vi "DCPowerlaw4i.vi"() -> ()   [LabVIEW 2011]
panel:
  in  "Temperature Array (K)":dbl[](array[numeric])=[6.0, 7.0, 8.0, 9.0, 10.0, 11.0] format="%#_6p"
  in  "Most Negative Voltage [V]":dbl=-5.0 format="%#.7p"
  in  "Voltage Step [V] 2":dbl=0.01 format="%#_7p"
  in  "Most Positive Voltage [V] 2":dbl=5.0 format="%#.7p"
  out "Temperature [K]":dbl
  out "V vs. Freq. 2":cluster{"Y":dbl[], "Y":dbl[]}[](graph)
  out "V vs. Freq.":cluster{"Y":dbl[], "Y":dbl[]}[](graph)
  in  "Voltage Step [V]":dbl=0.01 format="%#_7p"
  in  "Most Positive Voltage [V]":dbl=5.0 format="%#.7p"
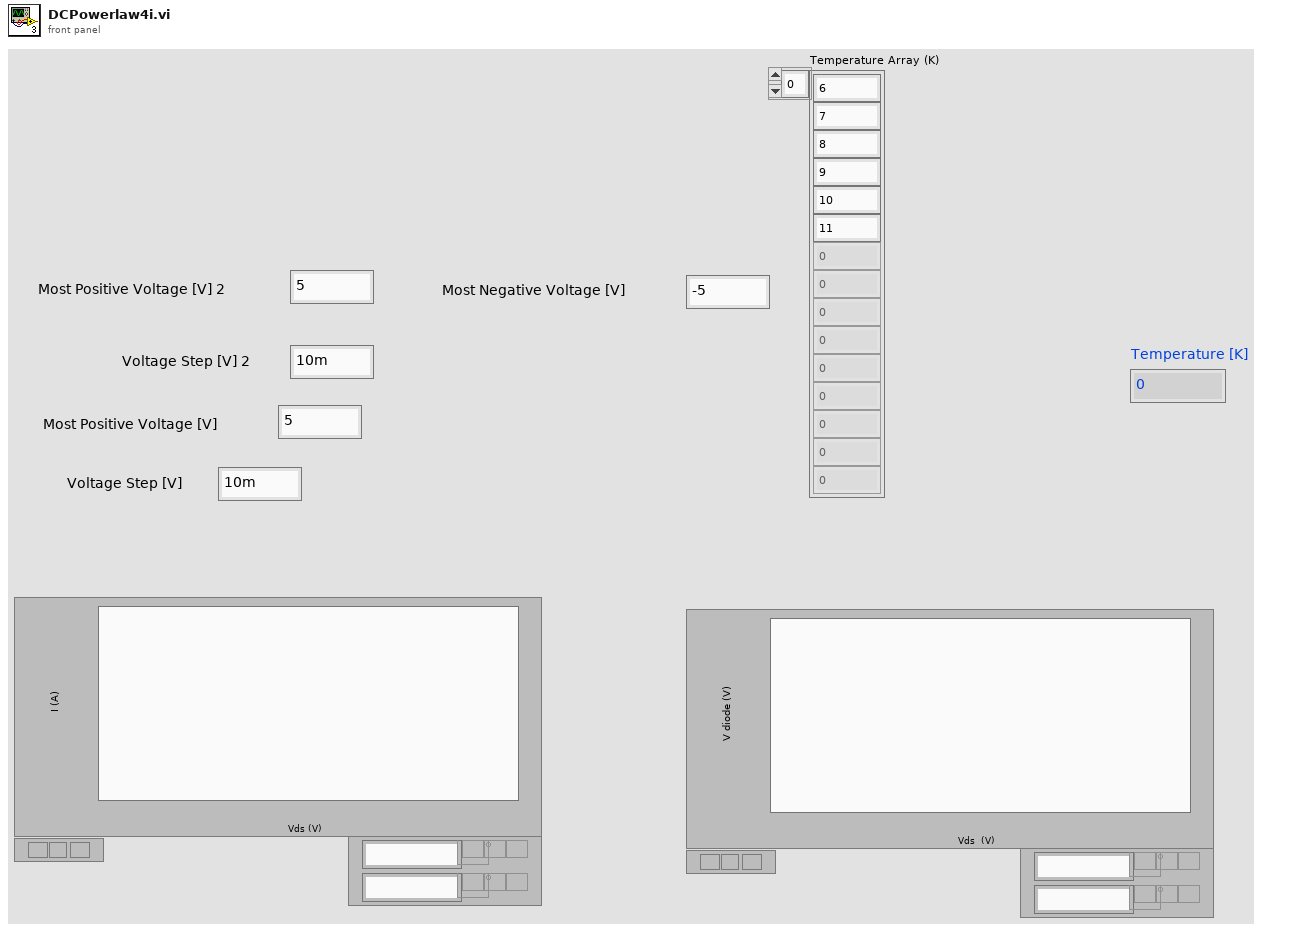
[diagram p1: front panel]
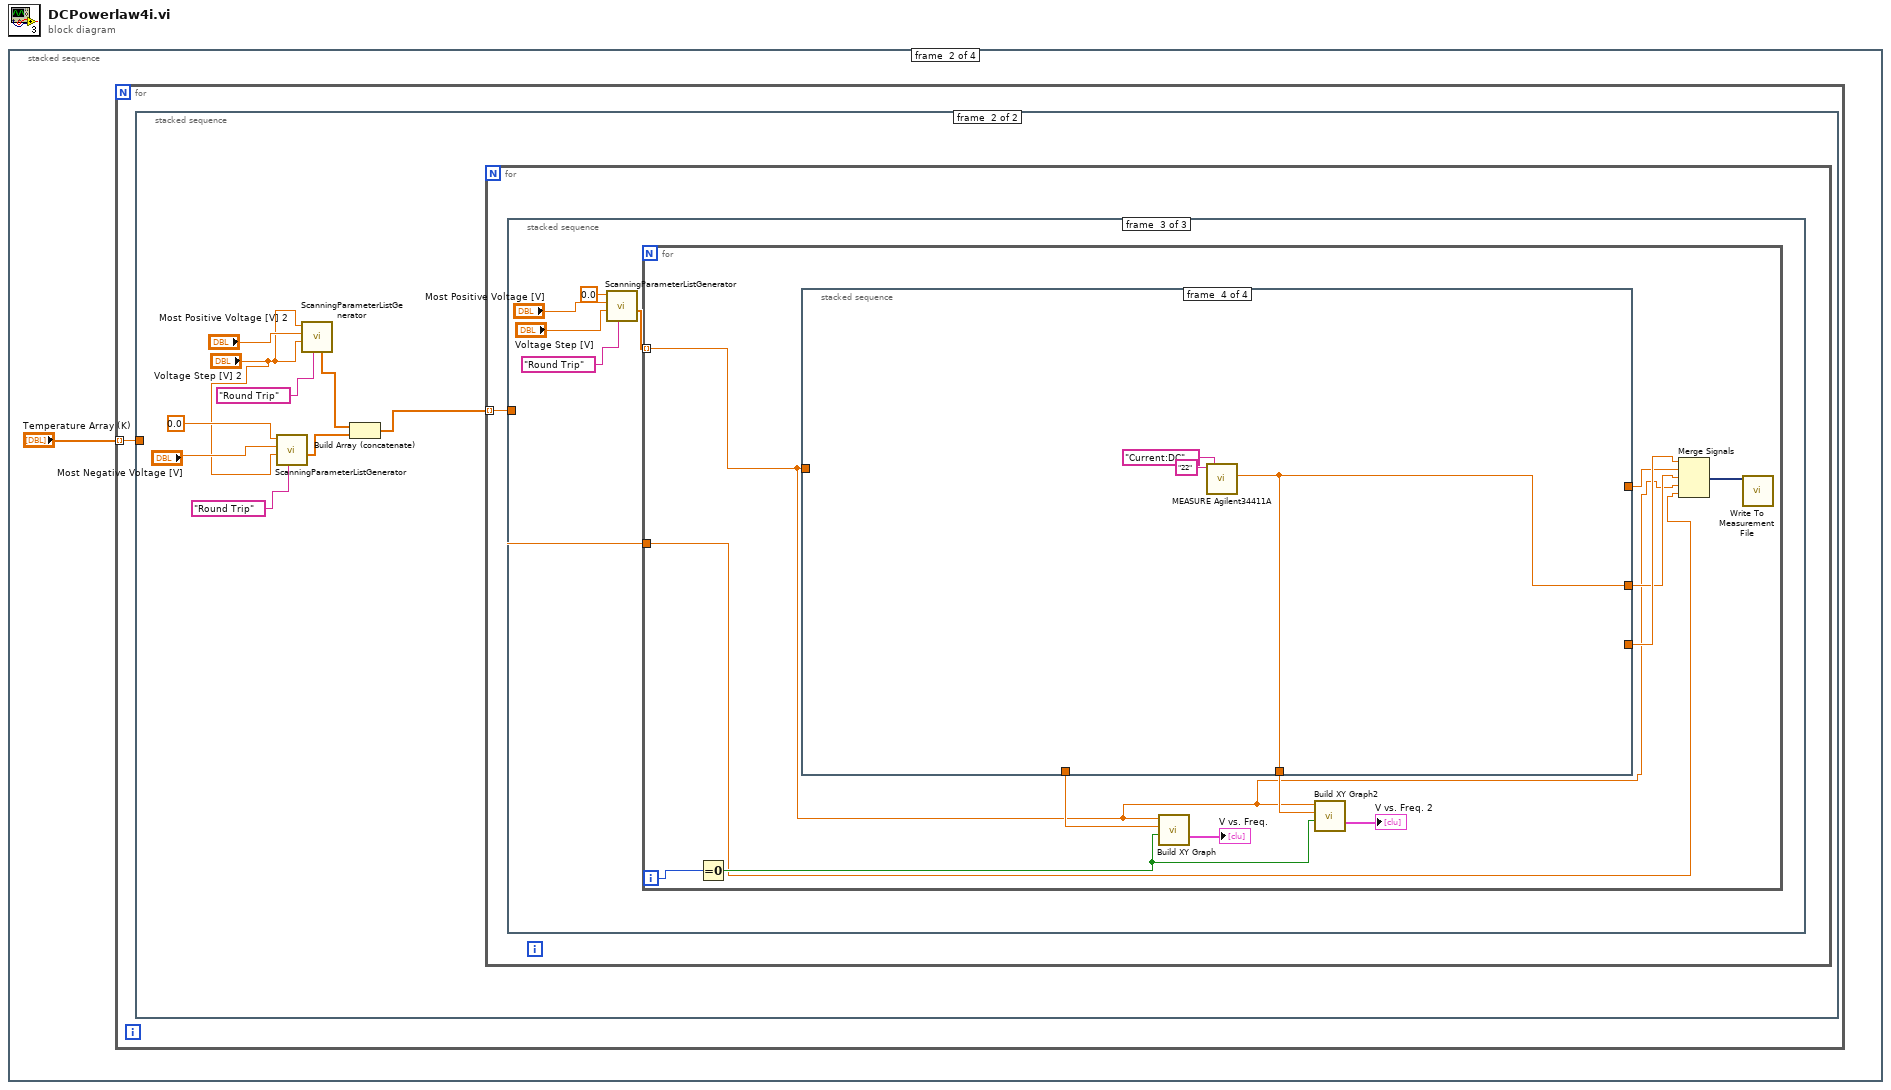
[diagram p0: block diagram]
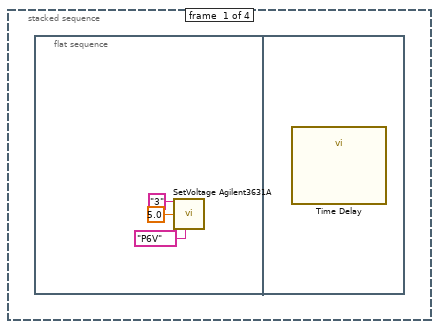
[diagram p2: hidden frame]
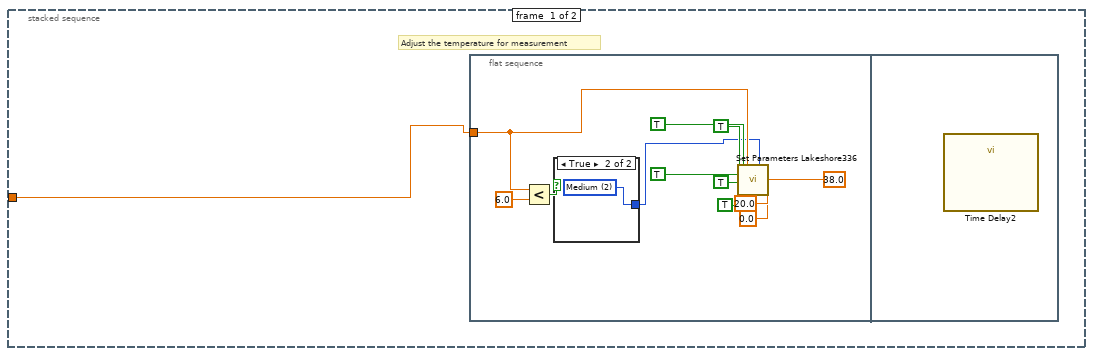
[diagram p3: hidden frame]
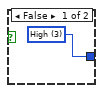
[diagram p4: hidden frame]
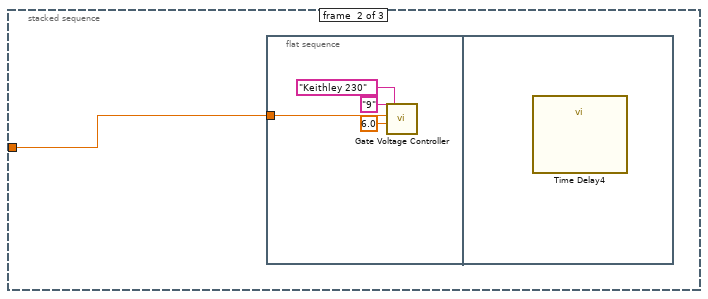
[diagram p6: hidden frame]
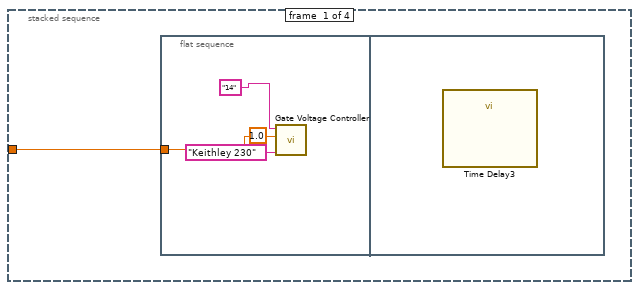
[diagram p7: hidden frame]
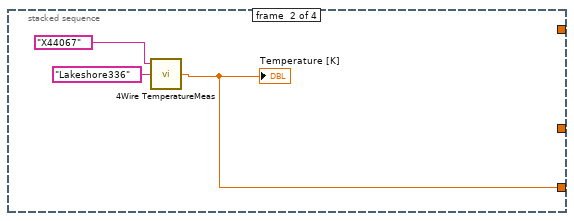
[diagram p8: hidden frame]
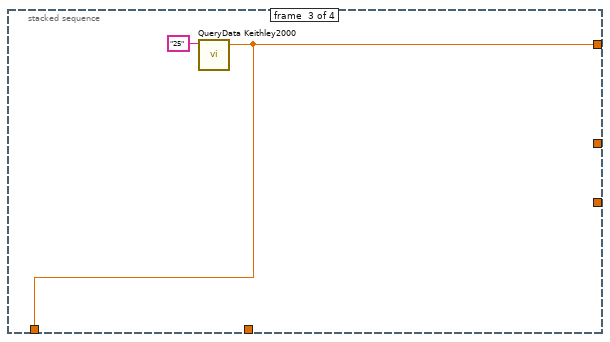
[diagram p9: hidden frame]
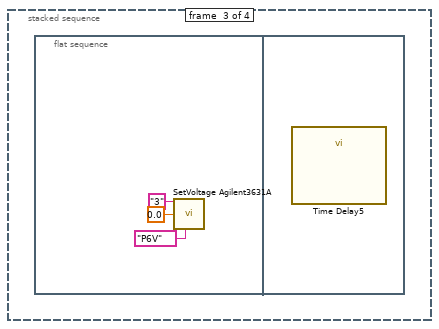
[diagram p10: hidden frame]
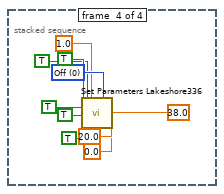
[diagram p11: hidden frame]
diagram:
  n1 = stacked-sequence {
    frame #0 {
      n2 = flat-sequence {
        frame #0 {
          n3 = call <userlib>:"SetVoltage Agilent3631A.vi"("address string"="3", "Voltage [V]"=5.0, "Channel"="P6V") -> ()  [unwired: 6 in]
        }
        frame #1 {
          n4 = call "Time Delay"() -> ()  [unwired: 11 in, 1 out]
        }
      }
    }
    frame #1 {
      n5 = for {
        tunnel: "Temperature Array (K)" -> [w5] mode=indexing
        n6 = stacked-sequence {
          tunnel: w5 -> [w6 _]
          frame #0 {
            # "Adjust the temperature for measurement"
            n7 = flat-sequence {
              tunnel: w6 -> [w10]
              frame #0 {
                n8 = Less?(x=w10, y=6.0) -> (x < y?=w8:bool)
                n9 = case shown="True" w8 {
                  tunnel: [w19 w20] -> w7
                  frame False {
                    w19 = u16 3 items=["High"=3, "Medium"=2, "Low (On)"=1, "Off"=0] ("Range (0:Off)")
                  }
                  frame True {
                    w20 = u16 2 items=["High"=3, "Medium"=2, "Low (On)"=1, "Off"=0] ("Range (0:Off)")
                  }
                }
                n10 = call <userlib>:"Set Parameters Lakeshore336.vi"("Write Gain?"=TRUE, "Write Int. Tc?"=TRUE, "Write Deri. Tc?"=TRUE, "Write Set Point?"=TRUE, "Set Point (K)"=w10, "Write Htr Range?"=TRUE, "Range (0:Off)"=w7, "Rate (D) (0.0 %)"=0.0, "Gain (P) (50.0)"=38.0, "Reset (I) (20.0)"=20.0) -> ()  [unwired: 13 in, 5 out]
              }
              frame #1 {
                n11 = call "Time Delay2"() -> ()  [unwired: 11 in, 1 out]
              }
            }
          }
          frame #1 {
            n12 = call <userlib>:"ScanningParameterListGenerator.vi"("Scanning Pattern"="Round Trip", "Step"="Voltage Step [V] 2", "Stop Value"="Most Negative Voltage [V]", "Start Value"=0.0 ("Stop Value")) -> ("Value List"=w25:dbl[])  [unwired: 6 in, 1 out]
            n13 = call <userlib>:"ScanningParameterListGenerator.vi"("Scanning Pattern"="Round Trip", "Step"="Voltage Step [V] 2", "Stop Value"="Most Positive Voltage [V] 2", "Start Value"="Voltage Step [V] 2") -> ("Value List"=w26:dbl[])  [unwired: 6 in, 1 out]
            n14 = Build Array (concatenate)(w26, w25) -> (w21:dbl[])
            n15 = for {
              tunnel: w21 -> [w30] mode=indexing
              n16 = stacked-sequence {
                tunnel: w30 -> [_ w31 w36]
                frame #0 {
                }
                frame #1 {
                  n17 = flat-sequence {
                    tunnel: w31 -> [w33]
                    frame #0 {
                      n18 = call <userlib>:"Gate Voltage Controller.vi"("Combo Box"="Keithley 230", "Theshold Voltage [V]"=6.0, "Set Voltage [V]"=w33, "address string"="9") -> ()  [unwired: 4 in]
                    }
                    frame #1 {
                      n19 = call "Time Delay4"() -> ()  [unwired: 11 in, 1 out]
                    }
                  }
                }
                frame #2 {
                  n20 = call <userlib>:"ScanningParameterListGenerator.vi"("Scanning Pattern"="Round Trip", "Step"="Voltage Step [V]", "Stop Value"="Most Positive Voltage [V]", "Start Value"=0.0) -> ("Value List"=w37:dbl[])  [unwired: 6 in, 1 out]
                  n21 = for {
                    tunnel: w37 -> [w43] mode=indexing
                    tunnel: w36 -> [w42]
                    i -> [w49]
                    n22 = Equal To 0?(x=w49) -> (x = 0?=w48:bool)
                    n23 = stacked-sequence {
                      tunnel: w43 -> [w54 _ _ _]
                      tunnel: [_ _ w62 _] -> w45
                      tunnel: [_ _ _ w64] -> w44
                      tunnel: [_ _ w62 _] -> w52
                      tunnel: [_ _ _ w64] -> w50
                      tunnel: [_ w59 _ _] -> w46
                      frame #0 {
                        n24 = flat-sequence {
                          tunnel: w54 -> [w57]
                          frame #0 {
                            n25 = call <userlib>:"Gate Voltage Controller.vi"("Combo Box"="Keithley 230", "Theshold Voltage [V]"=1.0, "Set Voltage [V]"=w57, "address string"="14") -> ()  [unwired: 4 in]
                          }
                          frame #1 {
                            n26 = call "Time Delay3"() -> ()  [unwired: 11 in, 1 out]
                          }
                        }
                      }
                      frame #1 {
                        n27 = call <userlib>:"4Wire TemperatureMeas.vi"("Instrument"="Lakeshore336", "Temperature Sensor"="X44067") -> ("Measured Temperature [K]"=w59:dbl)  [unwired: 2 in, 1 out]
                        "Temperature [K]" <- w59
                      }
                      frame #2 {
                        n28 = call <userlib>:"QueryData Keithley2000.vi"("address string"="25") -> ("value"=w62:dbl)  [unwired: 5 in]
                      }
                      frame #3 {
                        n29 = call <userlib>:"MEASURE Agilent34411A.vi"("Quantity"="Current:DC", "address string"="22") -> ("value"=w64:dbl)  [unwired: 5 in]
                      }
                    }
                    n30 = call "Build XY Graph"("Reset"=w48, "Y Input"=w52, "X Input"=w43) -> ("XY Graph"=→"V vs. Freq.":cluster{"Y":dbl[], "Y":dbl[]}[])  [unwired: 7 in, 1 out]
                    n31 = call "Build XY Graph2"("Reset"=w48, "Y Input"=w50, "X Input"=w43) -> ("XY Graph"=→"V vs. Freq. 2":cluster{"Y":dbl[], "Y":dbl[]}[])  [unwired: 7 in, 1 out]
                    n32 = Merge Signals(w46, w45, w44, w43, w42) -> (w47:dynamicdata)
                    n33 = call "Write To Measurement File"("Signals"=w47) -> ()  [unwired: 16 in, 3 out]
                  }
                }
              }
            }
          }
        }
      }
    }
    frame #2 {
      n34 = flat-sequence {
        frame #0 {
          n35 = call <userlib>:"SetVoltage Agilent3631A.vi"("address string"="3", "Voltage [V]"=0.0, "Channel"="P6V") -> ()  [unwired: 6 in]
        }
        frame #1 {
          n36 = call "Time Delay5"() -> ()  [unwired: 11 in, 1 out]
        }
      }
    }
    frame #3 {
      w79 = u16 0 items=["High"=3, "Medium"=2, "Low (On)"=1, "Off"=0] ("Range (0:Off)")
      n37 = call <userlib>:"Set Parameters Lakeshore336.vi"("Write Gain?"=TRUE, "Write Int. Tc?"=TRUE, "Write Deri. Tc?"=TRUE, "Write Set Point?"=TRUE, "Set Point (K)"=1.0, "Write Htr Range?"=TRUE, "Range (0:Off)"=w79, "Rate (D) (0.0 %)"=0.0, "Gain (P) (50.0)"=38.0, "Reset (I) (20.0)"=20.0) -> ()  [unwired: 13 in, 5 out]
    }
  }
